vi "switch_line_ERRADO.vi"(8 "Fault type":string="BC", 9 "Event type":string="SL", 10 "Fault time":string="045", 11 "Node fault":dbl) -> (3 "Result":string)   [LabVIEW 2019]
panel:
  # "SWITCH LINE"
  # "Nó virtual"
  # "nó virtual 2"
  # "SW_source"
  # "SW_load"
  # "Rs"
  # "Rl"
  # "N000VAS000NA       -1.       10.                                             0\n  N000VBS000NB       -1.       10.                                             0\n  N000VCS000NC       -1.       10.                                             0\n  S000NAN0025A       -1.       10.                                             0\n  S000NBN0025B       -1.       10.                                             0\n  S000NCN0025C       -1.       10.                                             0\n  S000NAS000ZA  0.125000       10.                                             0\n  S000NBS000ZB  0.125000       10.                                             0\n  S000NCS000ZC  0.125000       10.                                             0\n  S000GAN000GA  0.125000       10.                                             0\n  S000GBN000GB  0.125000       10.                                             0\n  S000GCN000GC  0.125000       10.                                             0"
  # "nó vitual para encaixar\na estrutura de chaves"
  # "S00Z1A\nS00Z1B\nS00Z1C"
  # "S00Z2A\nS00Z2B\nS00Z2C"
  # "N00__A\nN00__B\nN00__C"
  # "N000VA\nN000VB\nN000VC"
  # "S00Z1A\nS00Z1B\nS00Z1C"
  # "S000NA\nS000NB\nS000NC"
  # "S000NA\nS000NB\nS000NC"
  # "S00Z2A\nS00Z2B\nS00Z2C"
  # "nó do sistema\n(local de falta)"
  # "S000NA\nS000NB\nS000NC"
  # "S000ZA\nS000ZB\nS000ZC"
  # "SW_fault"
  # "S000ZA\nS000ZB\nS000ZC"
  # "S000PA\nS000PB\nS000PC"
  # "RLC"
  # "S000GA\nS000GB\nS000GC"
  # "S00Z3A\nS00Z3B\nS00Z3C"
  # "S000ZAS000GA            100.00                                               0\n  S000ZBS000GB            100.00                                               0\n  S000ZCS000GC            100.00                                               0\n  N000GA                   .0001                                               0\n  N000GB                   .0001                                               0\n  N000GC                   .0001                                               0"
  # "S00Z3A\nS00Z3B\nS00Z3C"
  # "SW_fault_G"
  # "S00Z3G"
  # "S00Z4G"
  # "-> curto"
  # "Rg"
  # "S00Z4G"
  # "Ground"
  # "S000PA\nS000PB\nS000PC"
  # "S000PA\nS000PC\nS000PA"
  # "SW_fault_phases"
  # "S000ZG"
  # "S00Z3G"
  # "Rz"
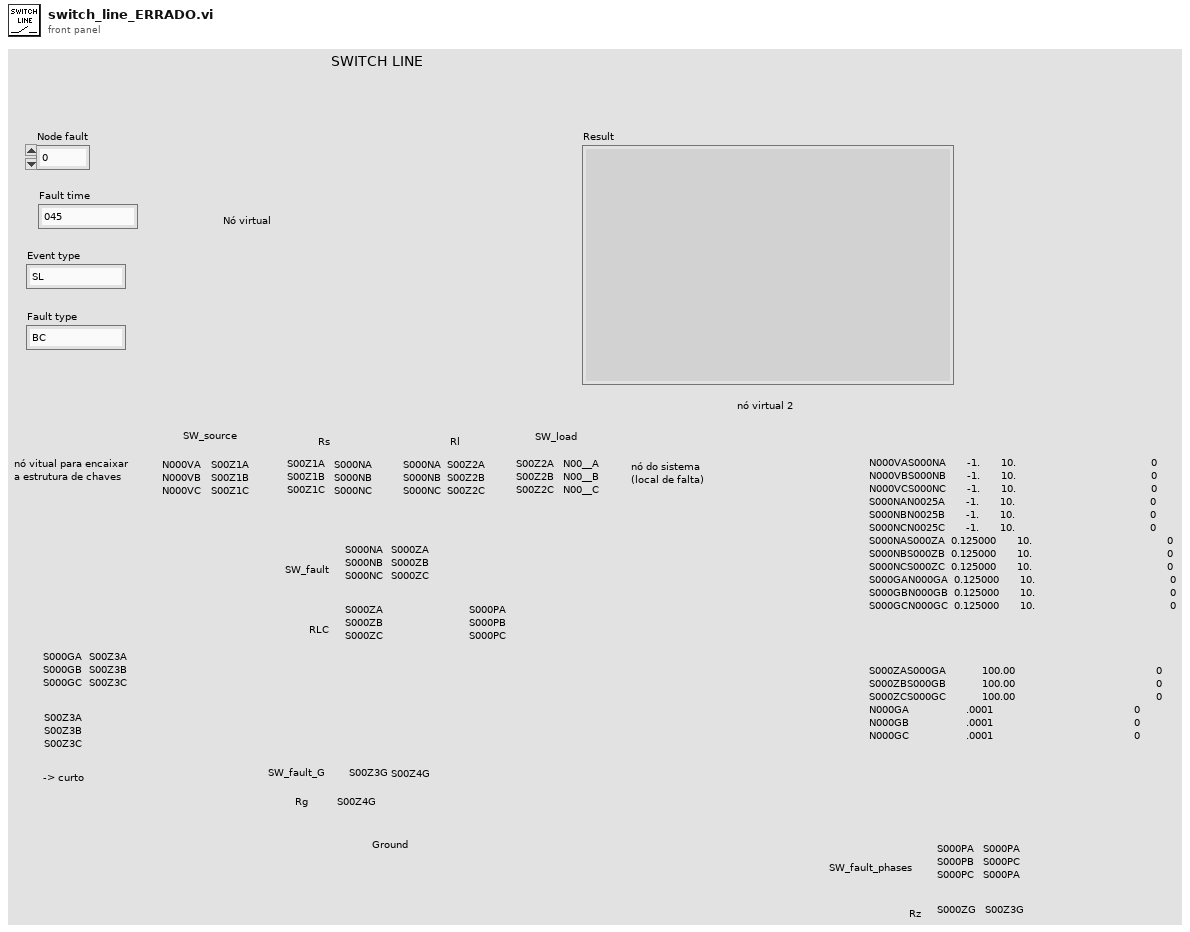
[diagram p1: front panel]
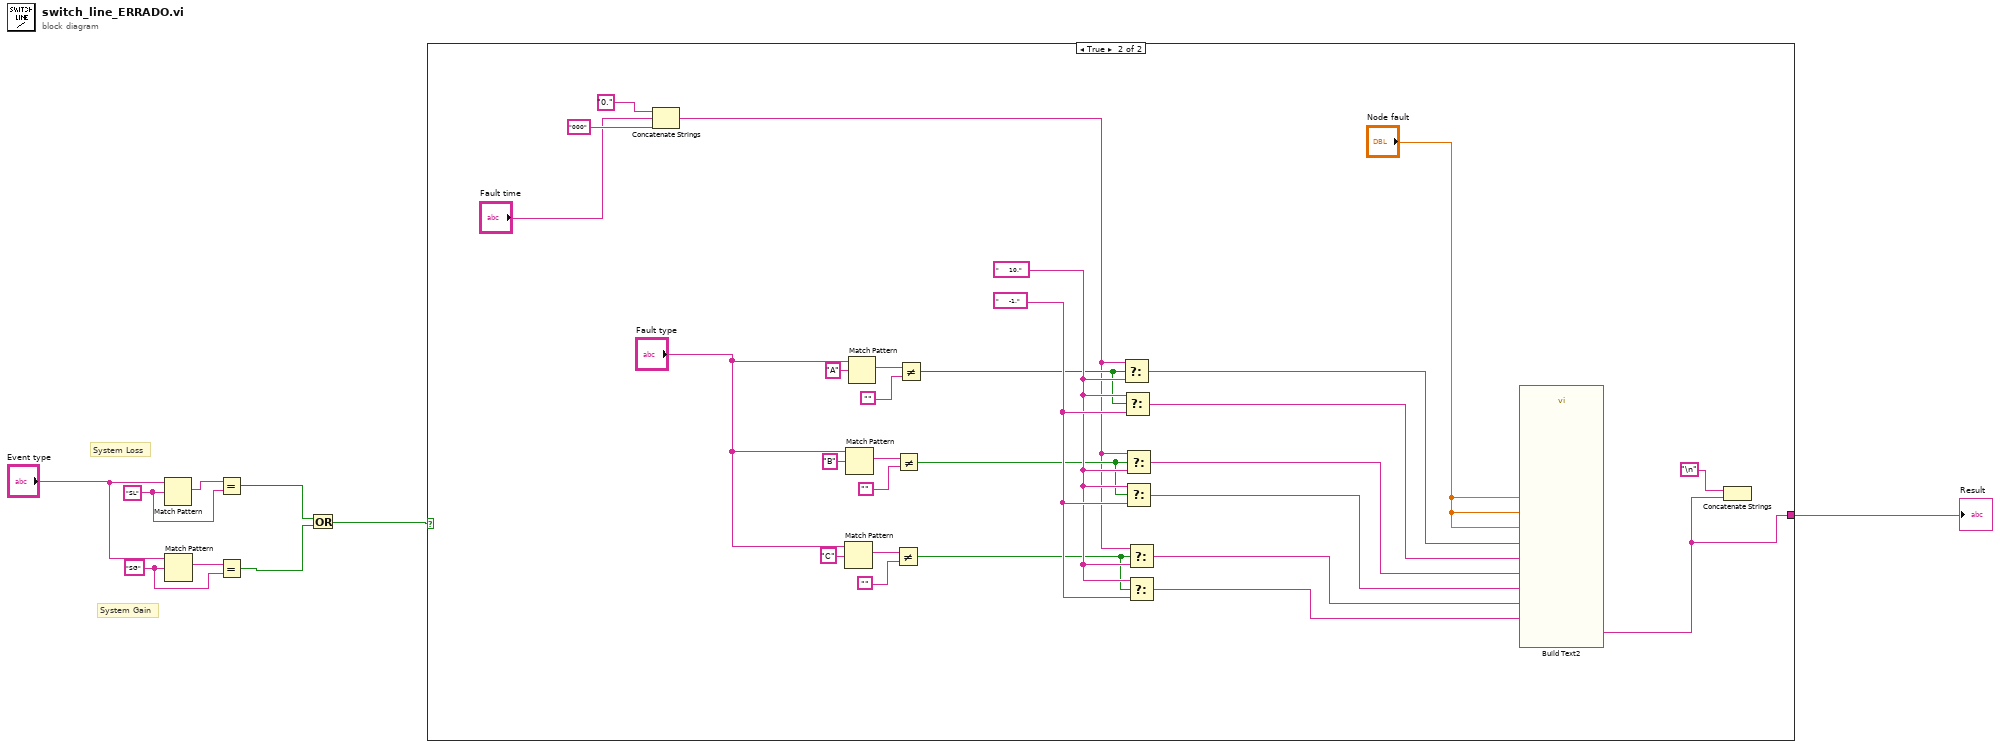
[diagram p0: block diagram]
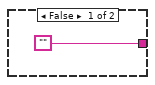
[diagram p2: hidden frame]
diagram:
  w7 = "SL" ("regular expression")
  w1 = "SG" ("regular expression")
  # "System Gain"
  # "System Loss"
  n1 = Match Pattern(string="Event type", regular expression=w7) -> (match substring=w6:string)  [unwired: 1 in, 3 out]
  n2 = Match Pattern(string="Event type", regular expression=w1) -> (match substring=w8:string)  [unwired: 1 in, 3 out]
  n3 = Equal?(x=w6, y=w7) -> (x = y?=w5:bool)
  n4 = Equal?(x=w8, y=w1) -> (x = y?=w4:bool)
  n5 = Or(x=w5, y=w4) -> (x .or. y?=w3:bool)
  n6 = case shown="True" w3 {
    tunnel: ["" w11] -> w9
    frame False {
    }
    frame True {
      w29 = "     -1."
      w27 = "     10."
      n7 = Concatenate Strings("0." ("string"), "Fault time", "000" ("string")) -> (w20:string)
      n8 = Match Pattern(string="Fault type", regular expression="C") -> (match substring=w31:string)  [unwired: 1 in, 3 out]
      n9 = Match Pattern(string="Fault type", regular expression="B") -> (match substring=w34:string)  [unwired: 1 in, 3 out]
      n10 = Match Pattern(string="Fault type", regular expression="A") -> (match substring=w37:string)  [unwired: 1 in, 3 out]
      n11 = Not Equal?(x=w31, y="") -> (x != y?=w24:bool)
      n12 = Not Equal?(x=w34, y="") -> (x != y?=w25:bool)
      n13 = Not Equal?(x=w37, y="") -> (x != y?=w26:bool)
      n14 = Select(t=w20, s=w26, f=w27) -> (s? t:f=w17:string)
      n15 = Select(t=w27, s=w26, f=w29) -> (s? t:f=w16:string)
      n16 = Select(t=w20, s=w25, f=w27) -> (s? t:f=w15:string)
      n17 = Select(t=w27, s=w25, f=w29) -> (s? t:f=w14:string)
      n18 = Select(t=w20, s=w24, f=w27) -> (s? t:f=w13:string)
      n19 = Select(t=w27, s=w24, f=w29) -> (s? t:f=w12:string)
      n20 = call "Build Text2"("outA"="Node fault", "time_close_A"=w17, "time_open_A"=w16, "outB"="Node fault", "time_close_B"=w15, "time_open_B"=w14, "outC"="Node fault", "time_close_C"=w13, "time_open_C"=w12) -> ("Result"=w11:string)  [unwired: 17 in, 1 out]
      n21 = Concatenate Strings("\n", w11) -> ()  [unwired: 1 out]
    }
  }
  "Result" <- w9
